vi "publisehr tests 1.vi"() -> ()   [LabVIEW 2018]
uses:
  publisher action.ctl
panel:
  in  "Boolean":bool
  out "number":dbl
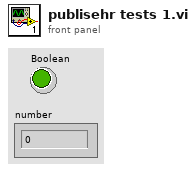
[diagram p1: front panel]
types:
  T1 = typedef "publisher action.ctl" = enum16{"set", "get", "init", "--send request", "--wait", "--respond", "init writer", "init reader"}
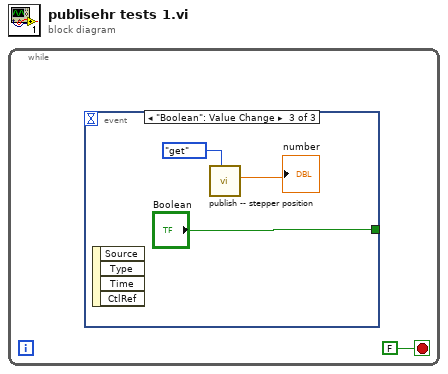
[diagram p0: block diagram]
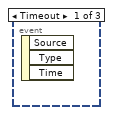
[diagram p2: hidden frame]
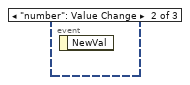
[diagram p3: hidden frame]
diagram:
  n1 = while {
    stop <- FALSE stop-if-true
    n2 = event shown="[2] \"Boolean\": Value Change" {
      selector: _ -> [_ _ _]
      dyn-events: _ -> [_ _ _]
      timeout: _ -> [_ _ _]
      tunnel: [_ _ "Boolean"] -> _
      event Timeout {
        n3 = event-data() -> ()  [unwired: 1 in, 3 out]
      }
      event "number": Value Change {
        n4 = event-data() -> ()  [unwired: 1 in, 1 out]
      }
      event "Boolean": Value Change {
        n5 = event-data() -> ()  [unwired: 1 in, 4 out]
        n6 = call "publish -- stepper position.vi"("publisher action"=publisher_action."get") -> ("stepper pos OUT"=→"number":dbl)  [unwired: 10 in]
      }
    }
  }
